vi "SetSimulatedFreq.vi"(8 "error in (no error)":errorcluster, 9 "Phase offset (deg)":dbl, 10 "Mixer freq [MHz]":dbl, 11 "Scope5785_six_channel":refnum<class "Scope5782_six_channel.lvclass">) -> (0 "error out":errorcluster, 3 "Scope5785_six_channel out":refnum<class "Scope5782_six_channel.lvclass">)   [LabVIEW 2018, in "Scope5782_six_channel.lvclass"]
uses:
  Scope5782_six_channel.lvclass
  Scope5782_six_channel.lvclass/Scope5782_six_channel.ctl
  <vilib>/Utility/error.llb/Error Cluster From Error Code.vi
  <vilib>/rvi/errors/niLvFpgaAdjustHostInterfaceError.vi
  <vilib>/rvi/interface/nirviReadWriteControl/nirviReadWriteControl.xnode
  FpgaRef/FpgaRefBase/Common FPGA ref.ctl
  FpgaRef/FpgaRef5761/FpgaRef5761.lvclass
  FpgaRef/FpgaRef5782/FpgaRef5782.lvclass
  NiFpgaLv.dll
  <vilib>/rvi/interface/Simulation/niFpgaSimulationCallBeginRW.vi
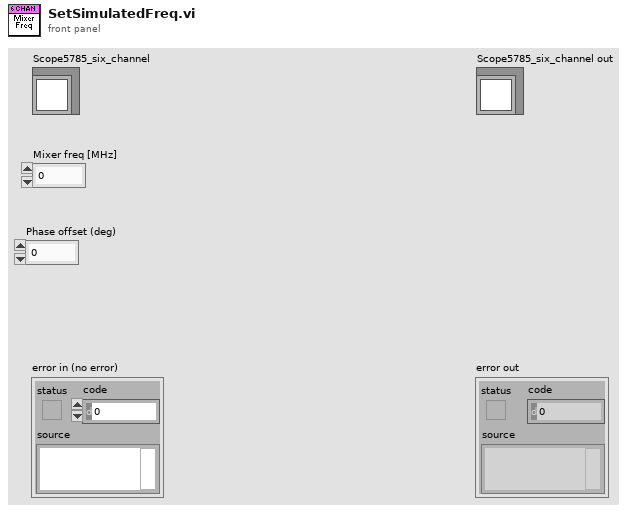
[diagram p1: front panel]
types:
  T1 = typedef "Common FPGA ref.ctl" = refnum<k20>
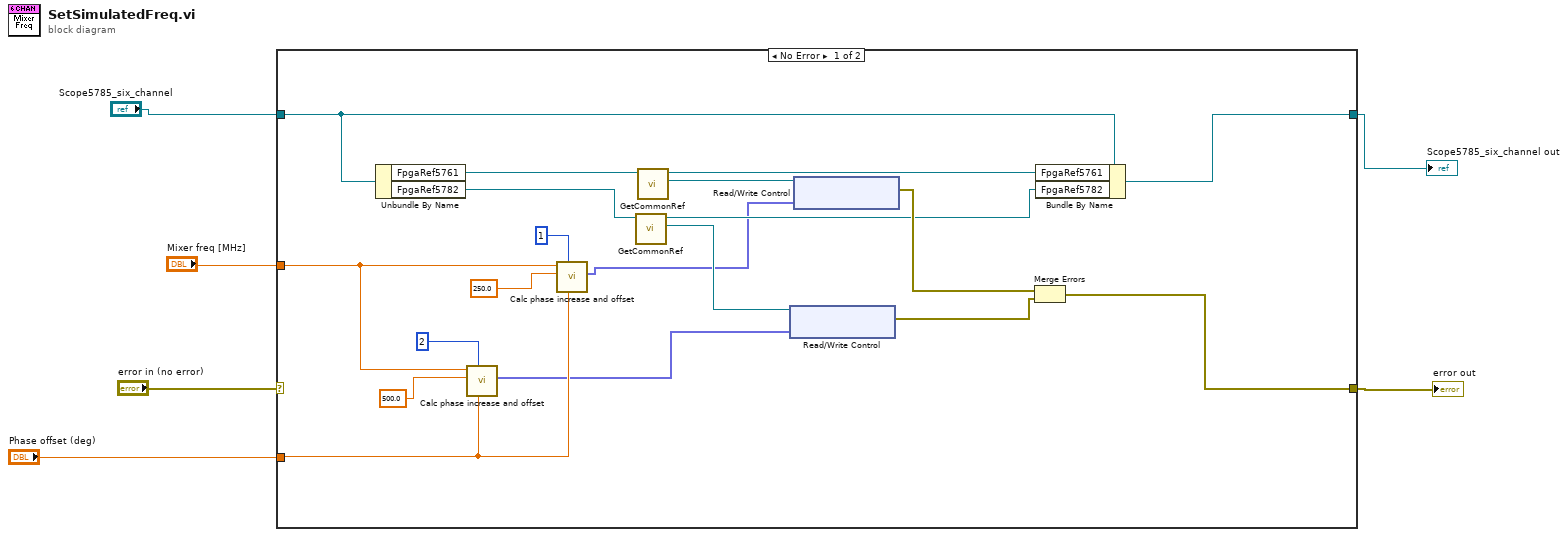
[diagram p0: block diagram]
diagram:
  n1 = case shown="No Error" "error in (no error)" {
    selector: "error in (no error)" -> [_ w26]
    tunnel: [w19 w26] -> w4
    tunnel: [w23 w25] -> w3
    tunnel: "Scope5785_six_channel" -> [w24 w25]
    tunnel: "Mixer freq [MHz]" -> [w11 _]
    tunnel: "Phase offset (deg)" -> [w10 _]
    frame No Error {
      n2 = Unbundle By Name(w24) -> ("FpgaRef5761"=w15:refnum<class "FpgaRef5761.lvclass">, "FpgaRef5782"=w17:refnum<class "FpgaRef5782.lvclass">)
      n3 = call "Calc phase increase and offset.vi"("Phase offset (deg)"=w10, "# of DDS"=2, "fclk (MHz)"=500.0 ("fclk (800MHz)"), "f_generated (MHz)"=w11) -> ("Phase out"=w7:fxp<+,64,64>[])  [unwired: 5 in, 2 out]
      n4 = call "Calc phase increase and offset.vi"("Phase offset (deg)"=w10, "# of DDS"=1, "fclk (MHz)"=250.0 ("fclk (800MHz)"), "f_generated (MHz)"=w11) -> ("Phase out"=w12:fxp<+,64,64>[])  [unwired: 5 in, 2 out]
      n5 = call-dynamic "GetCommonRef.vi"("FpgaRef5782 In"=w17) -> ("Common ref"=w14:T1, "FpgaRef5782 Out"=w16:refnum<class "FpgaRef5782.lvclass">)  [unwired: 8 in, 1 out]
      n6 = call-dynamic "GetCommonRef.vi"("FpgaRef5761 in"=w15) -> ("Common ref"=w18:T1)  [unwired: 8 in, 2 out]
      n7 = xnode "Read/Write Control"("FPGA VI Reference In"=w14, "Simulated phase"=w7) -> ("error out"=w13:errorcluster)  [unwired: 1 in, 1 out]
      n8 = xnode "Read/Write Control"("FPGA VI Reference In"=w18, "Simulated phase"=w12) -> ("error out"=w20:errorcluster)  [unwired: 1 in, 1 out]
      n9 = Merge Errors(w20, w13) -> (w19:errorcluster)
      n10 = Bundle By Name(cluster=w24, "FpgaRef5761"=w15, "FpgaRef5782"=w16) -> (w23:refnum<class "Scope5782_six_channel.lvclass">)
    }
    frame Error {
    }
  }
  "error out" <- w4
  "Scope5785_six_channel out" <- w3
